vi "task3.vi"() -> ()   [LabVIEW 2017]
panel:
  in  "stop":bool
  out "Thermometer":dbl(slide) scale=0.0..255.0
  in  "Array":bool[](array[boolean])
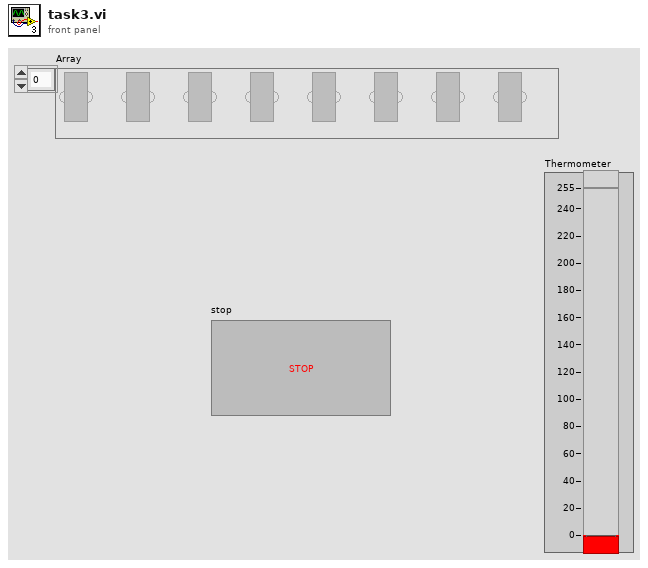
[diagram p1: front panel]
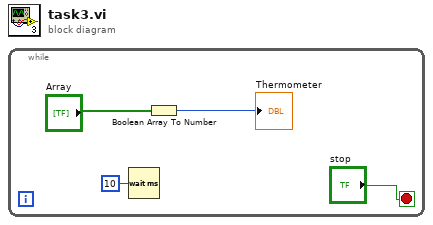
[diagram p0: block diagram]
diagram:
  n1 = while {
    stop <- "stop" stop-if-true
    n2 = Wait (ms)(milliseconds to wait=u32 10) -> ()  [unwired: 1 out]
    n3 = Boolean Array To Number(Boolean array="Array") -> (number=→"Thermometer":u32)
  }
